vi "STBY_MESSEN.vi"(0 "Standby":bool, 5 "Messen":bool, 7 "Case Nr.":i32, 11 "error in (no error)":errorcluster caption="Fehler (Eingang, kein Fehler)", 13 "Aktion":T1) -> (4 "Standby":bool, 6 "Messen":bool, 8 "Case Nr.":i32, 15 "error out":errorcluster caption="Fehler (Ausgang)")   [LabVIEW 2020, in "ABB-EL3000.lvlib" / "FID.lvlib"]
uses:
  FID.lvlib
  Aktion STY_MES.ctl
panel:
  # "0.....Initialisieren\n1.....Modbus lesen\n2.....Modbus schreiben"
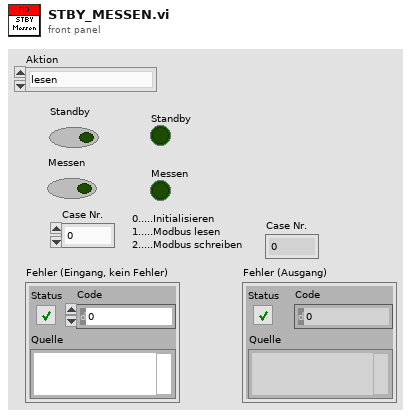
[diagram p1: front panel]
types:
  T1 = typedef "Aktion STY_MES.ctl" = enum16{"lesen", "setze STY", "setze MES", "MODBUS schreiben"}
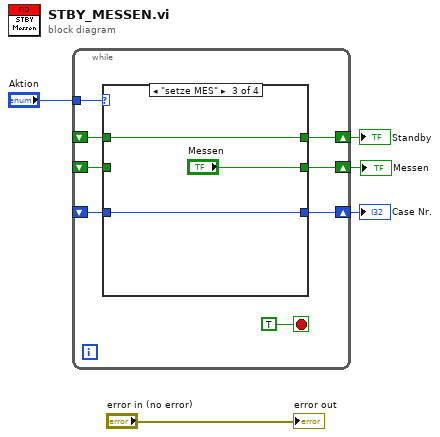
[diagram p0: block diagram]
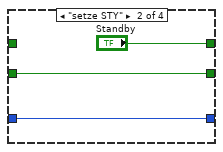
[diagram p3: hidden frame]
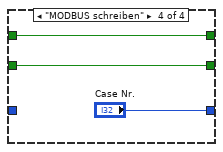
[diagram p4: hidden frame]
diagram:
  n1 = while {
    tunnel: "Aktion" -> [w12]
    shift-right: [w11] -> w4
    shift-left: _ -> [w10]
    shift-right: [w9] -> w3
    shift-left: _ -> [w8]
    shift-right: [w7] -> w2
    shift-left: _ -> [w6]
    stop <- TRUE stop-if-true
    n2 = case shown="\"setze MES\"" w12 {
      tunnel: [w16 "Standby" w21 w25] -> w11
      tunnel: w10 -> [w16 _ w21 w25]
      tunnel: [w15 w18 "Messen" w24] -> w9
      tunnel: w8 -> [w15 w18 _ w24]
      tunnel: [w14 w17 w20 "Case Nr."] -> w7
      tunnel: w6 -> [w14 w17 w20 _]
      frame "lesen", Default {
      }
      frame "setze STY" {
      }
      frame "setze MES" {
      }
      frame "MODBUS schreiben" {
      }
    }
  }
  "Standby" <- w4
  "Messen" <- w3
  "Case Nr." <- w2
  "error out" <- "error in (no error)"
